vi "Marker Types.vi"() -> (1 "Close":bool=TRUE, 3 "Type":T1=enum."vert")   [LabVIEW 2014, in "Graph Extensions.lvlib"]
uses:
  Graph Extensions.lvlib
  <vilib>/Utility/miscctls.llb/LVRectTypeDef.ctl
  controls/Simple Global for Marker Options.vi
  controls/markerType.ctl
  controls/cmd_options.ctl
  controls/commands.ctl
  controls/GraphExt-Cmds.ctl
  <vilib>/Utility/miscctls.llb/LVPoint32TypeDef.ctl
  <vilib>/Utility/inputDevices.llb/mouseAcquire.vi
panel:
  out "ClickedType":T1=enum."vert"
  in  "Close":bool
  in  "Tab Control":enum32{"Type", "Options", "Edit"}(tab)
  in  "Arrow":bool
  in  "Point":bool
  in  "Horizontal Line":bool
  in  "Verticle Line":bool
  in  "Verticle Range":bool
  in  "Horizontal Range":bool
  in  "Box Range":bool
  in  "Color":u32(colorbox)
  in  "Size":i16=14 min=4 max=72
  in  "Marker Color":u32(colorbox)
  in  "Style":T2(ring)
  in  "Width":u16=2 min=1 max=8
  in  "Remove":bool
  in  "Y2":dbl
  in  "Y1":dbl
  in  "X2":dbl
  in  "X1":dbl
  in  "Type":T1
  in  "Name":string
  in  "Listbox":i32(listbox)
  # "Marker"
  # "Font"
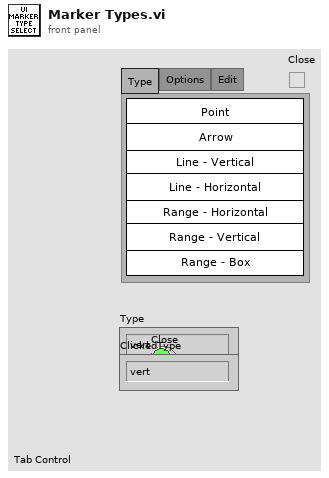
[diagram p1: front panel]
types:
  T1 = typedef "Graph Extensions.lvlib/markerType.ctl" = enum16{"point", "arrow", "horiz", "vert", "vert range", "horiz range", "box"}
  T2 = enum32{"Solid", "Dash", "Dot", "DashDot", "DashDotDot"}
  T3 = typedef "LVRectTypeDef.ctl" = cluster{"Left":i16, "Top":i16, "Right":i16, "Bottom":i16}
  T4 = typedef "Graph Extensions.lvlib/MarkerOptions.ctl" = cluster{"Color":u32, "pen":cluster{"Width":u16, "Style":enum32{"Solid", "Dash", "Dot", "DashDot", "DashDotDot"}}, "font":cluster{"Font Name":string, "Size":i16, "Strikeout?":bool, "Italic?":bool, "Underline?":bool, "Outline?":bool, "Shadow?":bool, "Bold?":bool, "FontColor":u32}, "caption":string}
  T5 = cluster{"Horizontal":i32, "Vertical":i32, "Scrolling":i32}
  T6 = typedef "Graph Extensions.lvlib/MarkerInfo.ctl" = cluster{"Type":T1, "X":dbl, "Y":dbl, "X2":dbl, "Y2":dbl, "Text":string}
  T7 = typedef "Graph Extensions.lvlib/cmd_options.ctl" = cluster{"Marker Color":u32, "Style":enum32{"Solid", "Dash", "Dot", "DashDot", "DashDotDot"}, "Width":u16, "Size":i16, "Color":u32}
  T8 = typedef "Graph Extensions.lvlib/commands.ctl" = enum16{"up", "options", "click", "move", "type", "redraw", "edited", "exit"}
  T9 = typedef "Graph Extensions.lvlib/GraphExt-Cmds.ctl" = cluster{"cmd":T8, "Type":T1, "Coords":T10, "text":string}
  T10 = typedef "LVPoint32TypeDef.ctl" = cluster{"Horizontal":i32, "Vertical":i32}
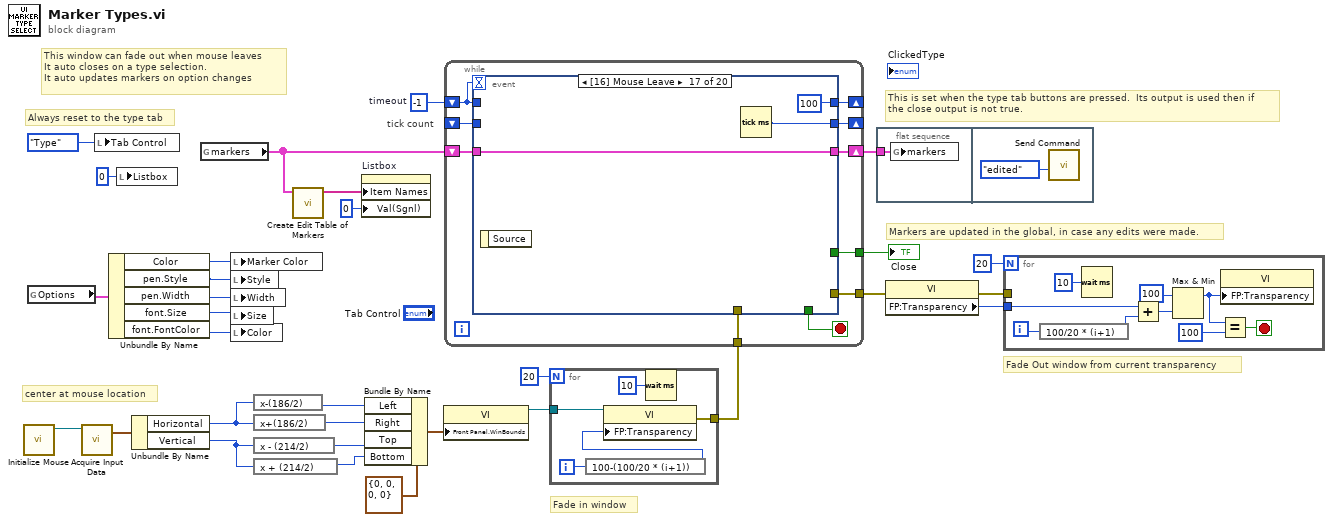
[diagram p0: block diagram]
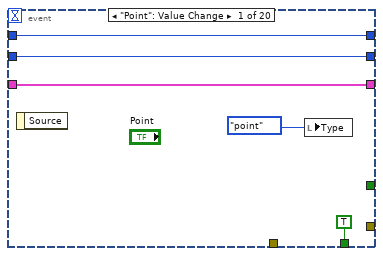
[diagram p2: hidden frame]
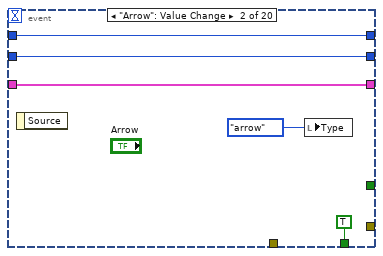
[diagram p3: hidden frame]
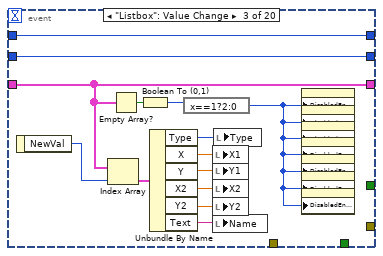
[diagram p4: hidden frame]
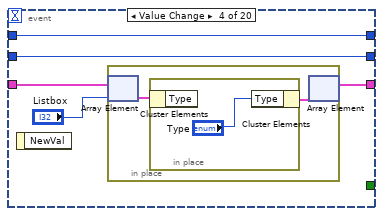
[diagram p5: hidden frame]
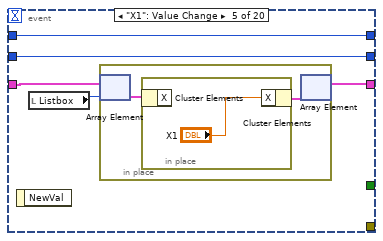
[diagram p6: hidden frame]
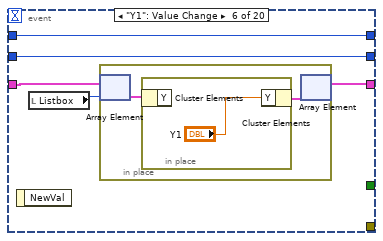
[diagram p7: hidden frame]
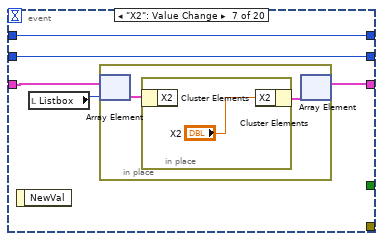
[diagram p8: hidden frame]
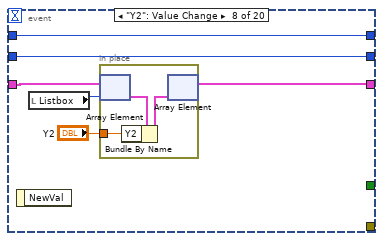
[diagram p9: hidden frame]
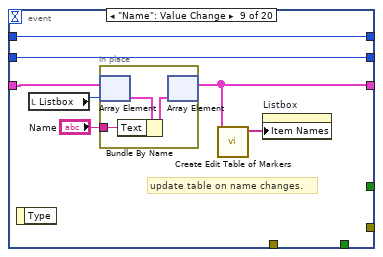
[diagram p10: hidden frame]
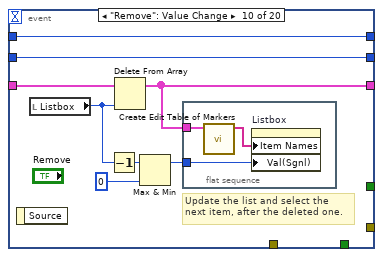
[diagram p11: hidden frame]
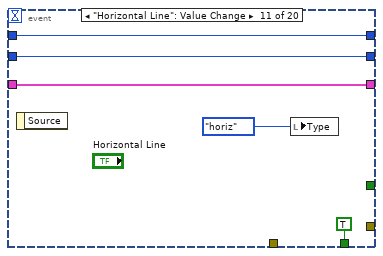
[diagram p12: hidden frame]
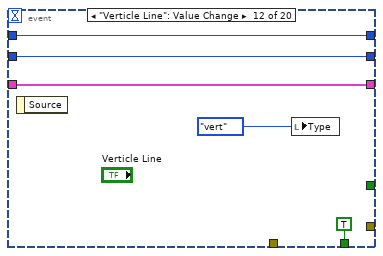
[diagram p13: hidden frame]
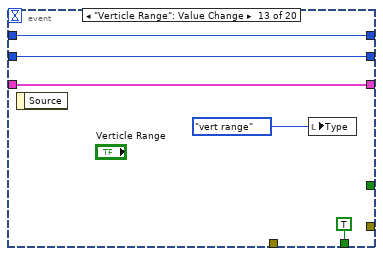
[diagram p14: hidden frame]
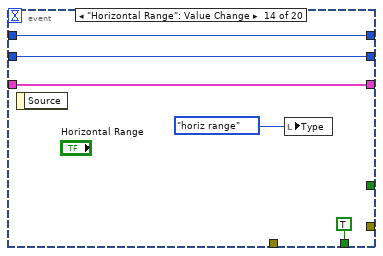
[diagram p15: hidden frame]
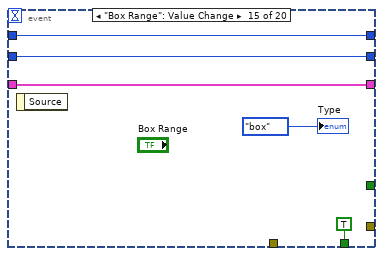
[diagram p16: hidden frame]
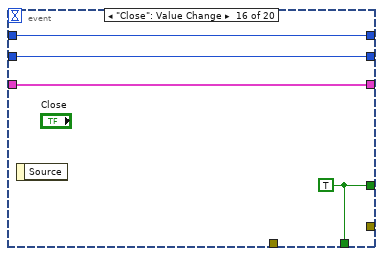
[diagram p17: hidden frame]
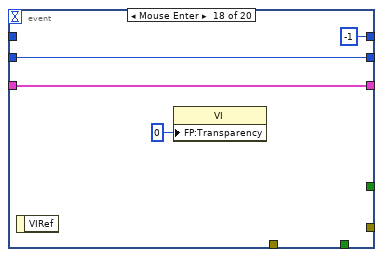
[diagram p18: hidden frame]
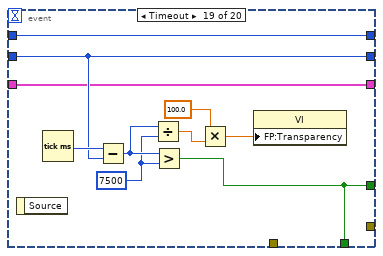
[diagram p19: hidden frame]
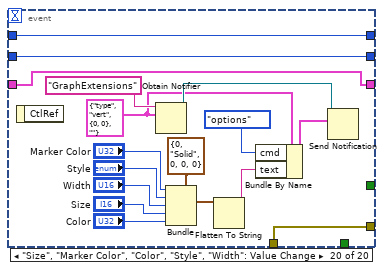
[diagram p20: hidden frame]
diagram:
  w13 = -1  # timeout
  # "Markers are updated in the global, in case any edits were made."
  # "This is set when the type tab buttons are pressed.  Its output is used then if\nthe close output is not true."
  # "This window can fade out when mouse leaves\nIt auto closes on a type selection.\nIt auto updates markers on option changes"
  # "tick count"
  # "Always reset to the type tab"
  # "Fade Out window from current transparency"
  # "Fade in window"
  # "center at mouse location"
  n1 = call <vilib>:"Initialize Mouse.vi"() -> ("device ID"=w29:refnum<k1>)  [unwired: 10 in, 1 out]
  n2 = global read "Simple Global for Marker Options.vi" "Options"() -> (w9:T4)
  n3 = call-poly <vilib>:"Acquire Input Data.vi"("device ID"=w29) -> ("axis info"=w28:T5)  [unwired: 15 in, 3 out]
  n4 = local write "Tab Control"(enum32{"Type", "Options", "Edit"}."Type" ("Tab Control")) -> ()
  n5 = Unbundle By Name(w9) -> ("Color"=w8:u32, "pen.Style"=w7:T2, "pen.Width"=w6:u16, "font.Size"=w5:i16, "font.FontColor"=w4:u32)
  n6 = local write "Listbox"(0 ("Listbox")) -> ()
  n7 = Unbundle By Name(w28) -> ("Horizontal"=w21:i32, "Vertical"=w22:i32)
  n8 = global read "Simple Global for Marker Options.vi" "markers"() -> (w2:T6[])
  n9 = local write "Marker Color"(w8) -> ()
  n10 = local write "Style"(w7) -> ()
  n11 = local write "Width"(w6) -> ()
  n12 = local write "Size"(w5) -> ()
  n13 = local write "Color"(w4) -> ()
  n14 = expression code="x-(186/2)"(w21) -> (w25:i32)
  n15 = expression code="x+(186/2)"(w21) -> (w26:i32)
  n16 = expression code="x - (214/2)"(w22) -> (w24:i32)
  n17 = expression code="x + (214/2)"(w22) -> (w23:i32)
  n18 = call "Create Edit Table of Markers.vi"("markers"=w2) -> ("Array"=w31:string[])  [unwired: 10 in]
  n19 = property on="Listbox" class="LstBox (strict)"("Item Names"=w31, "Val(Sgnl)"=0 ("Value (Signaling)")) -> ()  [unwired: 2 in, 2 out]
  n20 = Bundle By Name(cluster=T3 {"Left"=0, "Top"=0, "Right"=0, "Bottom"=0} ("Front Panel Window:Window Bounds"), "Left"=w25, "Right"=w26, "Top"=w24, "Bottom"=w23) -> (w20:T3)
  n21 = property class="VI"("Front Panel.WinBounds"=w20) -> (reference out=w19:refnum<vi>)  [unwired: 2 in, 1 out]
  n22 = for {
    N: 20 -> [_]
    tunnel: w19 -> [w36]
    tunnel: [w32] -> w17
    i -> [w35]
    n23 = expression code="100-(100/20 * (i+1))"(w35) -> (w34:i32)
    n24 = property class="VI"(reference=w36, "FP:Transparency"=w34) -> (error out=w32:errorcluster)  [unwired: 1 in, 1 out]
    n25 = Wait (ms)(milliseconds to wait=u32 10) -> ()  [unwired: 1 out]
  }
  n26 = while {
    tunnel: w17 -> [w46]
    tunnel: [w45] -> w15
    shift-right: [w42] -> _
    shift-left: w13 -> [w43]
    shift-right: [w41] -> _
    shift-left: _ -> [w40]
    tunnel: [w39] -> w12
    shift-right: [w37] -> w1
    shift-left: w2 -> [w38]
    stop <- w44 stop-if-true
    n27 = event shown="[16] Mouse Leave" {
      selector: _ -> [_ _ _ _ _ _ _ _ _ _ _ _ _ _ _ _ _ _ _ _]
      dyn-events: _ -> [_ _ _ _ _ _ _ _ _ _ _ _ _ _ _ _ _ _ _ _]
      timeout: w43 -> [_ _ _ _ _ _ _ _ _ _ _ _ _ _ _ _ _ _ _ _]
      tunnel: [_ _ _ _ _ _ _ _ _ _ _ _ _ _ _ w161 _ _ w175 _] -> w45
      tunnel: w46 -> [_ _ _ _ _ _ _ _ _ _ _ _ _ _ _ _ _ _ _ w180]
      tunnel: [TRUE TRUE _ _ _ _ _ _ _ _ TRUE TRUE TRUE TRUE TRUE w161 _ _ w175 _] -> w44
      tunnel: w43 -> [w49 w54 w70 w75 w83 w91 w99 w108 w118 w129 w135 w140 w145 w150 w155 w160 _ _ w178 w182]
      tunnel: [w49 w54 w70 w75 w83 w91 w99 w108 w118 w129 w135 w140 w145 w150 w155 w160 100 -1 w178 w182] -> w42
      tunnel: [w48 w53 w69 w74 w82 w90 w98 w107 w117 w128 w134 w139 w144 w149 w154 w159 w163 w168 w176 w181] -> w41
      tunnel: w40 -> [w48 w53 w69 w74 w82 w90 w98 w107 w117 w128 w134 w139 w144 w149 w154 w159 _ w168 w176 w181]
      tunnel: [_ _ _ _ _ _ _ _ _ _ _ _ _ _ _ _ _ _ _ w180] -> w39
      tunnel: w38 -> [w47 w52 w61 w72 w81 w89 w97 w106 w116 w127 w133 w138 w143 w148 w153 w158 w162 w165 w169 w179]
      tunnel: [w47 w52 w61 w71 w80 w88 w96 w105 w112 w123 w133 w138 w143 w148 w153 w158 w162 w165 w169 w179] -> w37
      event "Point": Value Change {
        n28 = event-data() -> ()  [unwired: 1 in, 1 out]
        n29 = local write "Type"(markerType."point" ("Type")) -> ()
      }
      event "Arrow": Value Change {
        n30 = event-data() -> ()  [unwired: 1 in, 1 out]
        n31 = local write "Type"(markerType."arrow" ("Type")) -> ()
      }
      event "Listbox": Value Change {
        n32 = event-data() -> ("NewVal"=w63:i32)  [unwired: 1 in]
        n33 = Index Array(array=w61, index=w63) -> (element=w62:T6)
        n34 = Empty Array?(array=w61) -> (empty?=w60:bool)
        n35 = Boolean To (0,1)(Boolean=w60) -> (0, 1=w59:i16)
        n36 = Unbundle By Name(w62) -> ("Type"=w64:T1, "X"=w65:dbl, "Y"=w66:dbl, "X2"=w67:dbl, "Y2"=w68:dbl, "Text"=w57:string)
        n37 = expression code="x==1?2:0"(w59) -> (w58:i16)
        n38 = local write "X1"(w65) -> ()
        n39 = local write "Y1"(w66) -> ()
        n40 = local write "X2"(w67) -> ()
        n41 = local write "Y2"(w68) -> ()
        n42 = local write "Name"(w57) -> ()
        n43 = local write "Type"(w64) -> ()
        n44 = property on="Type" class="Enum (strict)"("DisabledEnum"=w58) -> ()  [unwired: 2 in, 2 out]
        n45 = property on="Remove" class="Bool"("DisabledEnum"=w58) -> ()  [unwired: 2 in, 2 out]
        n46 = property on="Y2" class="DigNum (strict)"("DisabledEnum"=w58) -> ()  [unwired: 2 in, 2 out]
        n47 = property on="Y1" class="DigNum (strict)"("DisabledEnum"=w58) -> ()  [unwired: 2 in, 2 out]
        n48 = property on="X2" class="DigNum (strict)"("DisabledEnum"=w58) -> ()  [unwired: 2 in, 2 out]
        n49 = property on="X1" class="DigNum (strict)"("DisabledEnum"=w58) -> ()  [unwired: 2 in, 2 out]
        n50 = property on="Name" class="Str"("DisabledEnum"=w58) -> ()  [unwired: 2 in, 2 out]
      }
      event Value Change {
        n51 = event-data() -> ()  [unwired: 1 in, 1 out]
        n52 = in-place {
          n53 = in-place-array #1(w72, "Listbox") -> (w77:T6)
          n54 = in-place {
            n55 = in-place-cluster #2(w77) -> ()  [unwired: 1 out]
            n56 = in-place-cluster #2("Type"="Type") -> (w76:T6)
          }
          n57 = in-place-array #1(w76) -> (w71:T6[])  [unwired: 1 out]
        }
      }
      event "X1": Value Change {
        n58 = event-data() -> ()  [unwired: 1 in, 1 out]
        n59 = local read "Listbox"() -> (w79:i32)
        n60 = in-place {
          n61 = in-place-array #3(w81, w79) -> (w85:T6)
          n62 = in-place {
            n63 = in-place-cluster #4(w85) -> ()  [unwired: 1 out]
            n64 = in-place-cluster #4("X"="X1") -> (w84:T6)
          }
          n65 = in-place-array #3(w84) -> (w80:T6[])  [unwired: 1 out]
        }
      }
      event "Y1": Value Change {
        n66 = event-data() -> ()  [unwired: 1 in, 1 out]
        n67 = local read "Listbox"() -> (w87:i32)
        n68 = in-place {
          n69 = in-place-array #5(w89, w87) -> (w93:T6)
          n70 = in-place {
            n71 = in-place-cluster #6(w93) -> ()  [unwired: 1 out]
            n72 = in-place-cluster #6("Y"="Y1") -> (w92:T6)
          }
          n73 = in-place-array #5(w92) -> (w88:T6[])  [unwired: 1 out]
        }
      }
      event "X2": Value Change {
        n74 = event-data() -> ()  [unwired: 1 in, 1 out]
        n75 = local read "Listbox"() -> (w95:i32)
        n76 = in-place {
          n77 = in-place-array #7(w97, w95) -> (w101:T6)
          n78 = in-place {
            n79 = in-place-cluster #8(w101) -> ()  [unwired: 1 out]
            n80 = in-place-cluster #8("X2"="X2") -> (w100:T6)
          }
          n81 = in-place-array #7(w100) -> (w96:T6[])  [unwired: 1 out]
        }
      }
      event "Y2": Value Change {
        n82 = event-data() -> ()  [unwired: 1 in, 1 out]
        n83 = local read "Listbox"() -> (w104:i32)
        n84 = in-place {
          in-place-border: "Y2" -> [w109]
          n85 = in-place-array #9(w106, w104) -> (w110:T6)
          n86 = Bundle By Name(cluster=w110, "Y2"=w109) -> (w111:T6)
          n87 = in-place-array #9(w111) -> (w105:T6[])  [unwired: 1 out]
        }
      }
      event "Name": Value Change {
        # "update table on name changes."
        n88 = event-data() -> ()  [unwired: 1 in, 1 out]
        n89 = local read "Listbox"() -> (w115:i32)
        n90 = in-place {
          in-place-border: "Name" -> [w119]
          n91 = in-place-array #10(w116, w115) -> (w121:T6)
          n92 = Bundle By Name(cluster=w121, "Text"=w119) -> (w120:T6)
          n93 = in-place-array #10(w120) -> (w112:T6[])  [unwired: 1 out]
        }
        n94 = call "Create Edit Table of Markers.vi"("markers"=w112) -> ("Array"=w114:string[])  [unwired: 10 in]
        n95 = property on="Listbox" class="LstBox (strict)"("Item Names"=w114) -> ()  [unwired: 2 in, 2 out]
      }
      event "Remove": Value Change {
        # "Update the list and select the \nnext item, after the deleted one."
        n96 = event-data() -> ()  [unwired: 1 in, 1 out]
        n97 = local read "Listbox"() -> (w124:i32)
        n98 = Decrement(x=w124) -> (x-1=w122:i32)
        n99 = Delete From Array(array=w127, index=w124) -> (array with subset deleted=w123:T6[])  [unwired: 1 in, 1 out]
        n100 = Max & Min(x=w122, y=0) -> (max(x,y)=w125:i32)  [unwired: 1 out]
        n101 = flat-sequence {
          tunnel: w125 -> [w132]
          tunnel: w123 -> [w131]
          frame #0 {
            n102 = call "Create Edit Table of Markers.vi"("markers"=w131) -> ("Array"=w130:string[])  [unwired: 10 in]
            n103 = property on="Listbox" class="LstBox (strict)"("Item Names"=w130, "Val(Sgnl)"=w132) -> ()  [unwired: 2 in, 2 out]
          }
        }
      }
      event "Horizontal Line": Value Change {
        n104 = event-data() -> ()  [unwired: 1 in, 1 out]
        n105 = local write "Type"(markerType."horiz" ("Type")) -> ()
      }
      event "Verticle Line": Value Change {
        n106 = event-data() -> ()  [unwired: 1 in, 1 out]
        n107 = local write "Type"(markerType."vert" ("Type")) -> ()
      }
      event "Verticle Range": Value Change {
        n108 = event-data() -> ()  [unwired: 1 in, 1 out]
        n109 = local write "Type"(markerType."vert range" ("Type")) -> ()
      }
      event "Horizontal Range": Value Change {
        n110 = event-data() -> ()  [unwired: 1 in, 1 out]
        n111 = local write "Type"(markerType."horiz range" ("Type")) -> ()
      }
      event "Box Range": Value Change {
        n112 = event-data() -> ()  [unwired: 1 in, 1 out]
        "Type" <- markerType."box" ("Type")
      }
      event "Close": Value Change {
        w161 = TRUE
        n113 = event-data() -> ()  [unwired: 1 in, 1 out]
      }
      event Mouse Leave {
        n114 = event-data() -> ()  [unwired: 1 in, 1 out]
        n115 = Tick Count (ms)() -> (millisecond timer value=w163:u32)
      }
      event Mouse Enter {
        n116 = event-data() -> ()  [unwired: 1 in, 1 out]
        n117 = property class="VI"("FP:Transparency"=u8 0 ("Front Panel Window:Transparency")) -> ()  [unwired: 2 in, 2 out]
      }
      event Timeout {
        w173 = u32 7500 ("y")
        n118 = event-data() -> ()  [unwired: 1 in, 1 out]
        n119 = Tick Count (ms)() -> (millisecond timer value=w177:u32)
        n120 = Subtract(x=w177, y=w176) -> (x-y=w174:u32)
        n121 = Divide(x=w174, y=w173) -> (x/y=w172:dbl)
        n122 = Greater?(x=w174, y=w173) -> (0:w175:bool)
        n123 = Multiply(x=100.0 ("y"), y=w172) -> (x*y=w171:dbl)
        n124 = property class="VI"("FP:Transparency"=w171) -> ()  [unwired: 2 in, 2 out]
      }
      event "Size", "Marker Color", "Color", "Style", "Width": Value Change {
        w191 = T9 {"cmd"=enum."type", "Type"=enum."vert", "Coords"={"Horizontal"=0, "Vertical"=0}, "text"=""}
        n125 = event-data() -> ()  [unwired: 1 in, 1 out]
        n126 = Obtain Notifier(name (unnamed)="GraphExtensions", notification data type=w191) -> (notifier out=w192:refnum<notifier>)  [unwired: 2 in, 2 out]
        n127 = Bundle(cluster=T7 {"Marker Color"=0, "Style"=enum."Solid", "Width"=0, "Size"=0, "Color"=0}, "Marker Color"="Marker Color", "Style"="Style", "Width"="Width", "Size"="Size", "Color"="Color") -> (w185:T7)
        n128 = Flatten To String(anything=w185) -> (data string=w184:string)  [unwired: 3 in, 2 out]
        n129 = Bundle By Name(cluster=w191, "cmd"=commands."options", "text"=w184) -> (w193:T9)
        n130 = Send Notification(notification=w193, notifier=w192) -> ()  [unwired: 1 in, 2 out]
      }
    }
  }
  "Close" <- w15
  n131 = flat-sequence {
    tunnel: w1 -> [w196]
    frame #0 {
      n132 = global write "Simple Global for Marker Options.vi" "markers"(w196) -> ()
    }
    frame #1 {
      n133 = call "Send Command.vi"("cmd"=commands."edited") -> ()  [unwired: 11 in]
    }
  }
  n134 = property class="VI"(error in=w12) -> (error out=w11:errorcluster, "FP:Transparency"=w10:u8)  [unwired: 1 in, 1 out]
  n135 = for {
    N: 20 -> [_]
    tunnel: w11 -> [_]
    tunnel: w10 -> [w199]
    i -> [w206]
    stop <- w200 stop-if-true
    n136 = expression code="100/20 * (i+1)"(w206) -> (w204:i32)
    n137 = Wait (ms)(milliseconds to wait=u32 10) -> ()  [unwired: 1 out]
    n138 = Add(x=w199, y=w204) -> (x+y=w203:i32)
    n139 = Max & Min(x=u32 100 ("milliseconds to wait"), y=w203) -> (max(x,y)=w201:u32)  [unwired: 1 out]
    n140 = Equal?(x=w201, y=u32 100 ("x")) -> (x = y?=w200:bool)
    n141 = property class="VI"("FP:Transparency"=w201) -> ()  [unwired: 2 in, 2 out]
  }
